vi "dual_picomotor_driver.vi"() -> ()   [LabVIEW 2018]
panel:
  in  "read position?":bool
  in  "move 1":bool
  in  "move 2":bool
  in  "zig zag delay (ms)":dbl=50.0 format="%#_13g"
  in  "zig zag iterations":i32=10
  in  "zig zag?":bool
  in  "Loop Timer (ms)":dbl=100.0 format="%#_13g"
  in  "stop controller?":bool
  in  "STOP MOTION?":bool
  out "Position Status 2":i32
  in  "relative move?":bool
  in  "Relative Steps 2":i32=-30
  in  "Motor 2":i32=2
  in  "Motor 1":i32=1
  in  "set zero?":bool
  out "Position Status 1":i32
  in  "Relative Steps 1":i32=-35
  out "error out":errorcluster
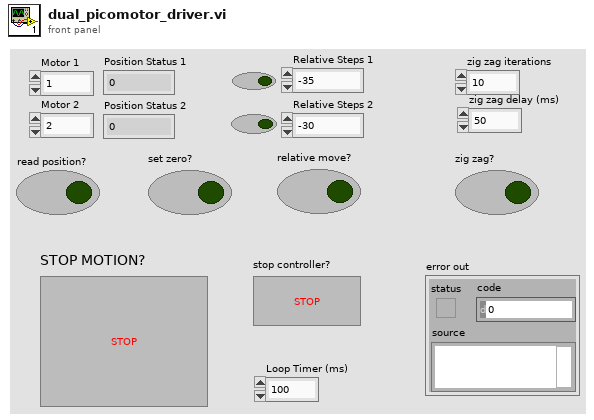
[diagram p1: front panel]
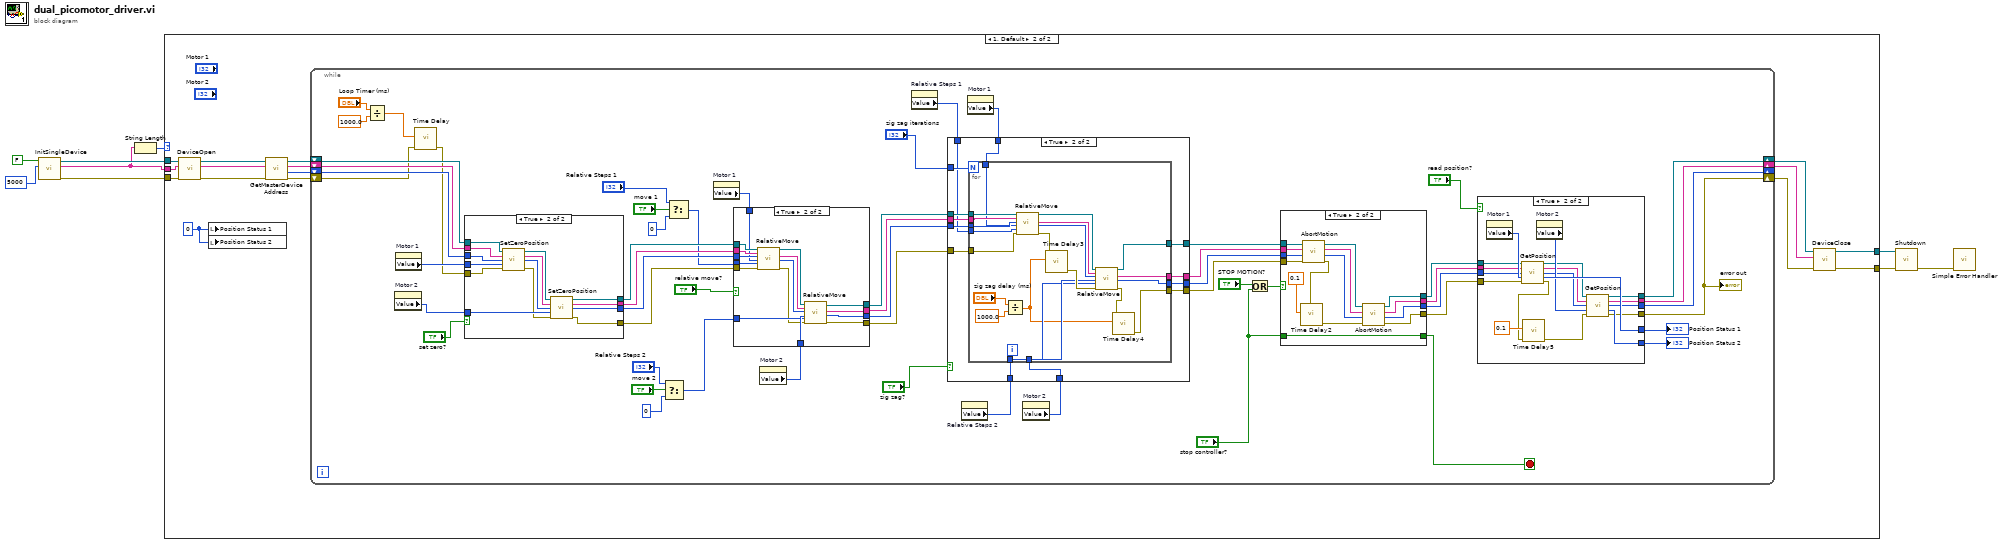
[diagram p0: block diagram]
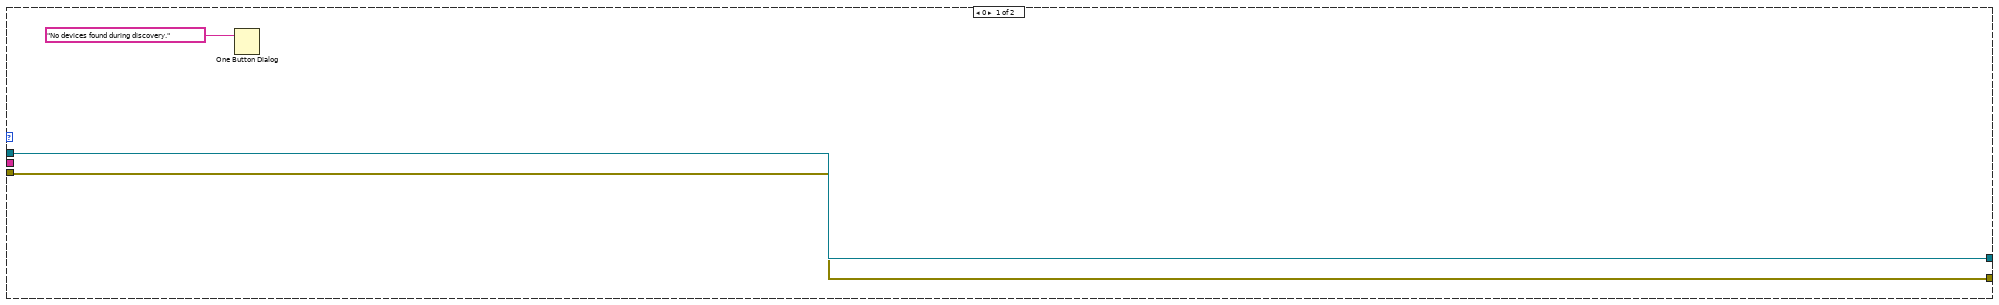
[diagram p2: hidden frame]
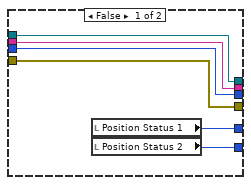
[diagram p3: hidden frame]
diagram:
  n1 = call "InitSingleDevice.vi"("msecDelayForDiscovery"=5000, "logging"=FALSE) -> ("error out"=w2:errorcluster, "DeviceKey Out"=w3:string, "CmdLib Out"=w5:refnum<k24>)  [unwired: 3 in]
  n2 = String Length(string=w3) -> (length=w4:i32)
  n3 = case shown="1, Default" w4 {
    tunnel: [w11 w21] -> w7
    tunnel: [w10 w22] -> w6
    tunnel: w5 -> [w11 w24]
    tunnel: w3 -> [_ w26]
    tunnel: w2 -> [w10 w28]
    frame 0 {
      n4 = One Button Dialog(message="No devices found during discovery.") -> ()  [unwired: 1 in, 1 out]
    }
    frame 1, Default {
      w13 = 0 ("Position Status 1")
      n5 = call "DeviceOpen.vi"("error in (no error)"=w28, "DeviceKey In"=w26, "CmdLib In"=w24) -> ("error out"=w27:errorcluster, "DeviceKey Out"=w25:string, "CmdLib Out"=w23:refnum<k24>)  [unwired: 2 in]
      n6 = local write "Position Status 1"(w13) -> ()
      n7 = local write "Position Status 2"(w13) -> ()
      n8 = call "GetMasterDeviceAddress.vi"("error in (no error)"=w27, "DeviceKey In"=w25, "CmdLib In"=w23) -> ("error out"=w20:errorcluster, "Device Address"=w19:i32, "DeviceKey Out"=w18:string, "CmdLib Out"=w17:refnum<k24>)  [unwired: 1 in]
      n9 = while {
        shift-right: [w55] -> w16
        shift-left: w17 -> [w80]
        shift-right: [w54] -> w15
        shift-left: w18 -> [w81]
        shift-right: [w53] -> _
        shift-left: w19 -> [w82]
        shift-right: [w29] -> w14
        shift-left: w20 -> [w69]
        stop <- w70 stop-if-true
        n10 = Divide(x="Loop Timer (ms)", y=1000.0) -> (x/y=w65:dbl)
        n11 = property on="Motor 2" class="DigNum (strict)"() -> ("Value"=w77:i32)  [unwired: 2 in, 2 out]
        n12 = property on="Motor 1" class="DigNum (strict)"() -> ("Value"=w78:i32)  [unwired: 2 in, 2 out]
        n13 = call "Time Delay"("error in (no error)"=w69, "Delay Time (s)"=w65) -> ("error out"=w68:errorcluster)  [unwired: 9 in]
        n14 = case shown="True" "set zero?" {
          tunnel: w78 -> [_ w203]
          tunnel: w77 -> [_ w202]
          tunnel: w68 -> [w189 w201]
          tunnel: w82 -> [w188 w200]
          tunnel: w81 -> [w187 w199]
          tunnel: w80 -> [w186 w198]
          tunnel: [w186 w197] -> w64
          tunnel: [w187 w196] -> w63
          tunnel: [w188 w195] -> w62
          tunnel: [w189 w194] -> w61
          frame False {
          }
          frame True {
            n15 = call <instrlib>:"SetZeroPosition.vi"("CmdLib In"=w198, "DeviceKey In"=w199, "Device Address In"=w200, "Motor"=w203, "error in (no error)"=w201) -> ("CmdLib Out"=w193:refnum<k24>, "DeviceKey Out"=w192:string, "Device Address Out"=w191:i32, "error out"=w190:errorcluster)  [unwired: 7 in]
            n16 = call <instrlib>:"SetZeroPosition.vi"("CmdLib In"=w193, "DeviceKey In"=w192, "Device Address In"=w191, "Motor"=w202, "error in (no error)"=w190) -> ("CmdLib Out"=w197:refnum<k24>, "DeviceKey Out"=w196:string, "Device Address Out"=w195:i32, "error out"=w194:errorcluster)  [unwired: 7 in]
          }
        }
        n17 = Select(t="Relative Steps 2", s="move 2", f=0) -> (s? t:f=w32:i32)
        n18 = Select(t="Relative Steps 1", s="move 1", f=0) -> (s? t:f=w37:i32)
        n19 = property on="Motor 1" class="DigNum (strict)"() -> ("Value"=w76:i32)  [unwired: 2 in, 2 out]
        n20 = property on="Motor 2" class="DigNum (strict)"() -> ("Value"=w75:i32)  [unwired: 2 in, 2 out]
        n21 = case shown="True" "relative move?" {
          tunnel: w37 -> [_ w185]
          tunnel: w32 -> [_ w174]
          tunnel: w64 -> [w169 w184]
          tunnel: w63 -> [w168 w183]
          tunnel: w62 -> [w167 w182]
          tunnel: w76 -> [_ w181]
          tunnel: w75 -> [_ w180]
          tunnel: w61 -> [w166 w179]
          tunnel: [w169 w178] -> w50
          tunnel: [w168 w177] -> w49
          tunnel: [w167 w176] -> w48
          tunnel: [w166 w175] -> w47
          frame False {
          }
          frame True {
            n22 = call "RelativeMove.vi"("CmdLib In"=w184, "DeviceKey In"=w183, "Device Address In"=w182, "Motor"=w181, "Relative Steps"=w185, "error in (no error)"=w179) -> ("CmdLib Out"=w173:refnum<k24>, "DeviceKey Out"=w172:string, "Device Address Out"=w171:i32, "error out"=w170:errorcluster)  [unwired: 10 in]
            n23 = call "RelativeMove.vi"("CmdLib In"=w173, "DeviceKey In"=w172, "Device Address In"=w171, "Motor"=w180, "Relative Steps"=w174, "error in (no error)"=w170) -> ("CmdLib Out"=w178:refnum<k24>, "DeviceKey Out"=w177:string, "Device Address Out"=w176:i32, "error out"=w175:errorcluster)  [unwired: 10 in]
          }
        }
        n24 = property on="Relative Steps 1" class="DigNum (strict)"() -> ("Value"=w44:i32)  [unwired: 2 in, 2 out]
        n25 = property on="Relative Steps 2" class="DigNum (strict)"() -> ("Value"=w43:i32)  [unwired: 2 in, 2 out]
        n26 = property on="Motor 1" class="DigNum (strict)"() -> ("Value"=w46:i32)  [unwired: 2 in, 2 out]
        n27 = property on="Motor 2" class="DigNum (strict)"() -> ("Value"=w45:i32)  [unwired: 2 in, 2 out]
        n28 = case shown="True" "zig zag?" {
          tunnel: "zig zag iterations" -> [_ w124]
          tunnel: w50 -> [w111 w123]
          tunnel: w49 -> [w110 w122]
          tunnel: w48 -> [w109 w121]
          tunnel: w47 -> [w108 w120]
          tunnel: w46 -> [_ w119]
          tunnel: w45 -> [_ w118]
          tunnel: w44 -> [_ w117]
          tunnel: w43 -> [_ w116]
          tunnel: [w111 w115] -> w42
          tunnel: [w110 w114] -> w41
          tunnel: [w109 w113] -> w40
          tunnel: [w108 w112] -> w39
          frame False {
          }
          frame True {
            n29 = for {
              N: w124 -> [_]
              tunnel: w123 -> [w140]
              tunnel: w122 -> [w139]
              tunnel: w121 -> [w138]
              tunnel: w120 -> [w137]
              tunnel: w119 -> [w136]
              tunnel: w118 -> [w135]
              tunnel: w117 -> [w134]
              tunnel: w116 -> [w133]
              tunnel: [w132] -> w115
              tunnel: [w131] -> w114
              tunnel: [w130] -> w113
              tunnel: [w128] -> w112
              n30 = Divide(x="zig zag delay (ms)", y=1000.0) -> (x/y=w125:dbl)
              n31 = call "RelativeMove.vi"("CmdLib In"=w140, "DeviceKey In"=w139, "Device Address In"=w138, "Motor"=w136, "Relative Steps"=w134, "error in (no error)"=w137) -> ("CmdLib Out"=w145:refnum<k24>, "DeviceKey Out"=w144:string, "Device Address Out"=w143:i32, "error out"=w142:errorcluster)  [unwired: 10 in]
              n32 = call "Time Delay3"("error in (no error)"=w142, "Delay Time (s)"=w125) -> ("error out"=w141:errorcluster)  [unwired: 9 in]
              n33 = call "RelativeMove.vi"("CmdLib In"=w145, "DeviceKey In"=w144, "Device Address In"=w143, "Motor"=w135, "Relative Steps"=w133, "error in (no error)"=w141) -> ("CmdLib Out"=w132:refnum<k24>, "DeviceKey Out"=w131:string, "Device Address Out"=w130:i32, "error out"=w129:errorcluster)  [unwired: 10 in]
              n34 = call "Time Delay4"("error in (no error)"=w129, "Delay Time (s)"=w125) -> ("error out"=w128:errorcluster)  [unwired: 9 in]
            }
          }
        }
        n35 = Or(x="STOP MOTION?", y="stop controller?") -> (x .or. y?=w71:bool)
        n36 = case shown="True" w71 {
          tunnel: w42 -> [w149 w154]
          tunnel: w41 -> [w148 w165]
          tunnel: w40 -> [w147 w164]
          tunnel: w39 -> [w146 w163]
          tunnel: [w150 w162] -> w70
          tunnel: "stop controller?" -> [w150 w162]
          tunnel: [w149 w161] -> w59
          tunnel: [w148 w160] -> w58
          tunnel: [w147 w159] -> w57
          tunnel: [w146 w158] -> w56
          frame False {
          }
          frame True {
            n37 = call <instrlib>:"AbortMotion.vi"("error in (no error)"=w163, "Device Address In"=w164, "DeviceKey In"=w165, "CmdLib In"=w154) -> ("error out"=w152:errorcluster, "Device Address Out"=w155:i32, "DeviceKey Out"=w156:string, "CmdLib Out"=w157:refnum<k24>)
            n38 = call "Time Delay2"("error in (no error)"=w152, "Delay Time (s)"=0.1) -> ("error out"=w151:errorcluster)  [unwired: 9 in]
            n39 = call <instrlib>:"AbortMotion.vi"("error in (no error)"=w151, "Device Address In"=w155, "DeviceKey In"=w156, "CmdLib In"=w157) -> ("error out"=w158:errorcluster, "Device Address Out"=w159:i32, "DeviceKey Out"=w160:string, "CmdLib Out"=w161:refnum<k24>)
          }
        }
        n40 = case shown="True" "read position?" {
          tunnel: [w84 w107] -> w74
          tunnel: [w85 w106] -> w73
          tunnel: w59 -> [w89 w103]
          tunnel: w58 -> [w88 w102]
          tunnel: w57 -> [w87 w101]
          tunnel: w56 -> [w86 w100]
          tunnel: [w89 w96] -> w55
          tunnel: [w88 w95] -> w54
          tunnel: [w87 w94] -> w53
          tunnel: [w86 w93] -> w29
          frame False {
            n41 = local read "Position Status 1"() -> (w85:i32)
            n42 = local read "Position Status 2"() -> (w84:i32)
          }
          frame True {
            n43 = property on="Motor 1" class="DigNum (strict)"() -> ("Value"=w105:i32)  [unwired: 2 in, 2 out]
            n44 = call <instrlib>:"GetPosition.vi"("CmdLib In"=w103, "DeviceKey In"=w102, "Device Address In"=w101, "Motor"=w105, "error in (no error)"=w100) -> ("CmdLib Out"=w99:refnum<k24>, "DeviceKey Out"=w98:string, "Device Address Out"=w97:i32, "Position"=w106:i32, "error out"=w90:errorcluster)  [unwired: 6 in]
            n45 = call "Time Delay5"("error in (no error)"=w90, "Delay Time (s)"=0.1) -> ("error out"=w91:errorcluster)  [unwired: 9 in]
            n46 = property on="Motor 2" class="DigNum (strict)"() -> ("Value"=w104:i32)  [unwired: 2 in, 2 out]
            n47 = call <instrlib>:"GetPosition.vi"("CmdLib In"=w99, "DeviceKey In"=w98, "Device Address In"=w97, "Motor"=w104, "error in (no error)"=w91) -> ("CmdLib Out"=w96:refnum<k24>, "DeviceKey Out"=w95:string, "Device Address Out"=w94:i32, "Position"=w107:i32, "error out"=w93:errorcluster)  [unwired: 6 in]
          }
        }
        "Position Status 2" <- w74
        "Position Status 1" <- w73
        "error out" <- w29
      }
      n48 = call "DeviceClose.vi"("error in (no error)"=w14, "DeviceKey In"=w15, "CmdLib In"=w16) -> ("error out"=w22:errorcluster, "CmdLib Out"=w21:refnum<k24>)  [unwired: 2 in, 1 out]
    }
  }
  n49 = call "Shutdown.vi"("error in (no error)"=w6, "CmdLib In"=w7) -> ("error out"=w1:errorcluster)  [unwired: 4 in, 1 out]
  n50 = call <vilib>:"Simple Error Handler.vi"("error in (no error)"=w1) -> ()  [unwired: 4 in, 5 out]
